vi "Controls-Loop.vi"(7 "CMD Notifier":refnum<notifier>, 8 "error in":errorcluster, 9 "Control Data Notifier":refnum<notifier>, 10 "Processed Data Notifier":refnum<notifier>, 11 "Message Queues":T2) -> (0 "error out":errorcluster)   [LabVIEW 2024]
uses:
  support/Message Queue/All Message Queues.ctl
  support/Message Queue/Message Cluster.ctl
  support/Control/Array Data Constant.ctl
  support/Control/Control Data Constant.ctl
  Controls State.ctl
  support/Control/DAQmx Container.ctl
  Sequence/Sequence Structure.ctl
  support/Control/BBControl Parameters.ctl
  support/Control/StreamCluster_TypeDef.ctl
  <vilib>/ErrorRing/Error Ring.xnode
  support/Message Queue/Message Queue.lvlib
  332b4253-326d-4d7b-9710-a01b345fab27.vi
  61c51413-b1d0-41cf-878e-839bc20d578b.vi
  c894b992-033a-4c8a-923e-e5ce24f73376.vi
panel:
  in  "Control Data":T1
  out "Loop-3 Iteration Clock (s) 2":dbl format="%10.8f"
  out "Loop-3 Iteration Counter 2":i32
  out "Loop-3 Iteration Counter":i32
  out "Loop-3 Iteration Clock (s)":dbl format="%10.8f"
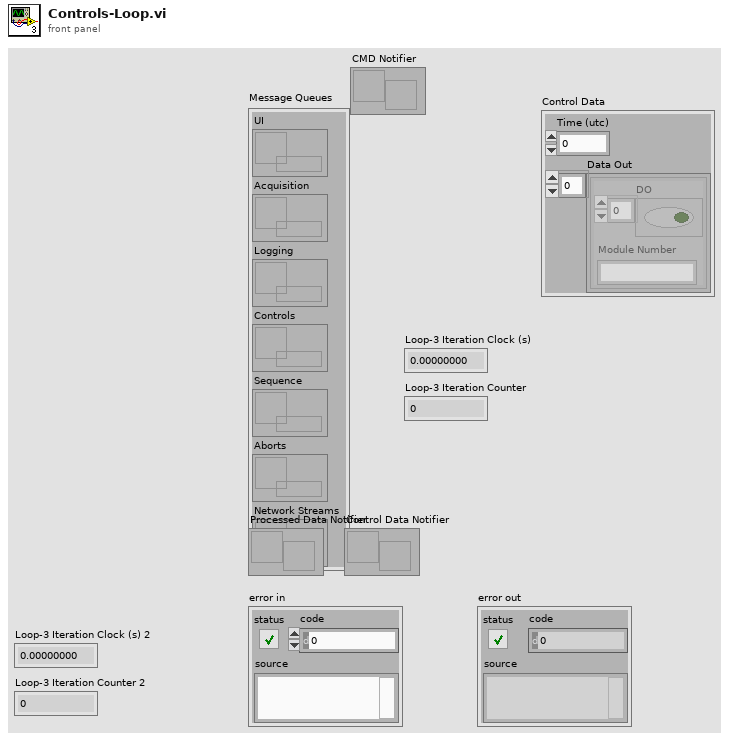
[diagram p1: front panel]
types:
  T1 = typedef "Control Data Constant.ctl" = cluster{"Time (utc)":ext, "Data Out":cluster{"DO":bool[], "Module Number":string}[]}
  T2 = typedef "Message Queue.lvlib/All Message Queues.ctl" = cluster{"UI":refnum<queue>, "Acquisition":refnum<queue>, "Logging":refnum<queue>, "Controls":refnum<queue>, "Sequence":refnum<queue>, "Aborts":refnum<queue>, "Network Streams":refnum<queue>}
  T3 = typedef "Controls State.ctl" = enum16{"Idle", "Control", "Sequencing", "Abort"}
  T4 = typedef "DAQmx Container.ctl" = cluster{"DAQmx Analog In":refnum<k21>, "DAQmx Digital In":refnum<k21>, "DAQmx Digital Out":refnum<k21>, "DAQmx Analog Out":refnum<k21>, "DAQmx 6343":refnum<k21>, "DAQmx IG-Sense":refnum<k21>, "DAQmx Thermo":refnum<k21>, "DAQmx Bridge":refnum<k21>, "DAQmx Trigger":refnum<k21>}
  T5 = typedef "LVDateTimeRec.ctl" = cluster{"fractional second":dbl, "second":i32, "minute":i32, "hour":i32, "day of month":i32, "month":i32, "year":i32, "day of week":i32, "day of year":i32, "DST":i32}
  T6 = typedef "BBControl Parameters.ctl" = cluster{"Sequence Delay (s)":dbl, "Sequence Duration (s)":dbl, "BBControl Criteria":cluster{"Channel Name":i32, "Comparison":u16, "Set":dbl, "Enabled":bool, "Valve Name":i32, "Upper":dbl, "Lower":dbl}[]}
  T7 = typedef "Sequence Structure.ctl" = cluster{"Sequence Controller":cluster{"Time (s)":dbl, "Enabled":bool, "Valve":u16[]}[], "Sequence Delay":dbl, "Sequence Duration":dbl}
  T8 = typedef "StreamCluster_TypeDef.ctl" = cluster{"DAQ":cluster{"ManagmentRate_Hz":i32, "StreamRate_Hz":i32, "StreamRate_ms":i32, "ManagmentRate_ms":i32, "refDesArray":cluster{"refDes-s":string[], "Module Number":string}[]}, "Modules":cluster{"Slot ID":i32, "Model Number":string, "Sample Rate s/S (Hz)":dbl, "Sensors":cluster{"refDes":string, "serialNumber":string, "modelNumber":string, "units":string, "balance":dbl, "sensitivity":dbl, "type":string, "inputTerminalConfiguration":string, "channelNumber":string, "taskName":string, "bridgeConfiguration":string, "excitationVoltage":dbl, "voltageExcitationSource":string, "nominalBridgeResistance":dbl, "firstElectricalValue":dbl, "secondElectricalValue":dbl, "firstPhysicalValue":dbl, "secondPhysicalValue":dbl, "electricalUnits":string}[]}[]}
  T9 = cluster{"refDes-s":string[], "Module Number":string}[]
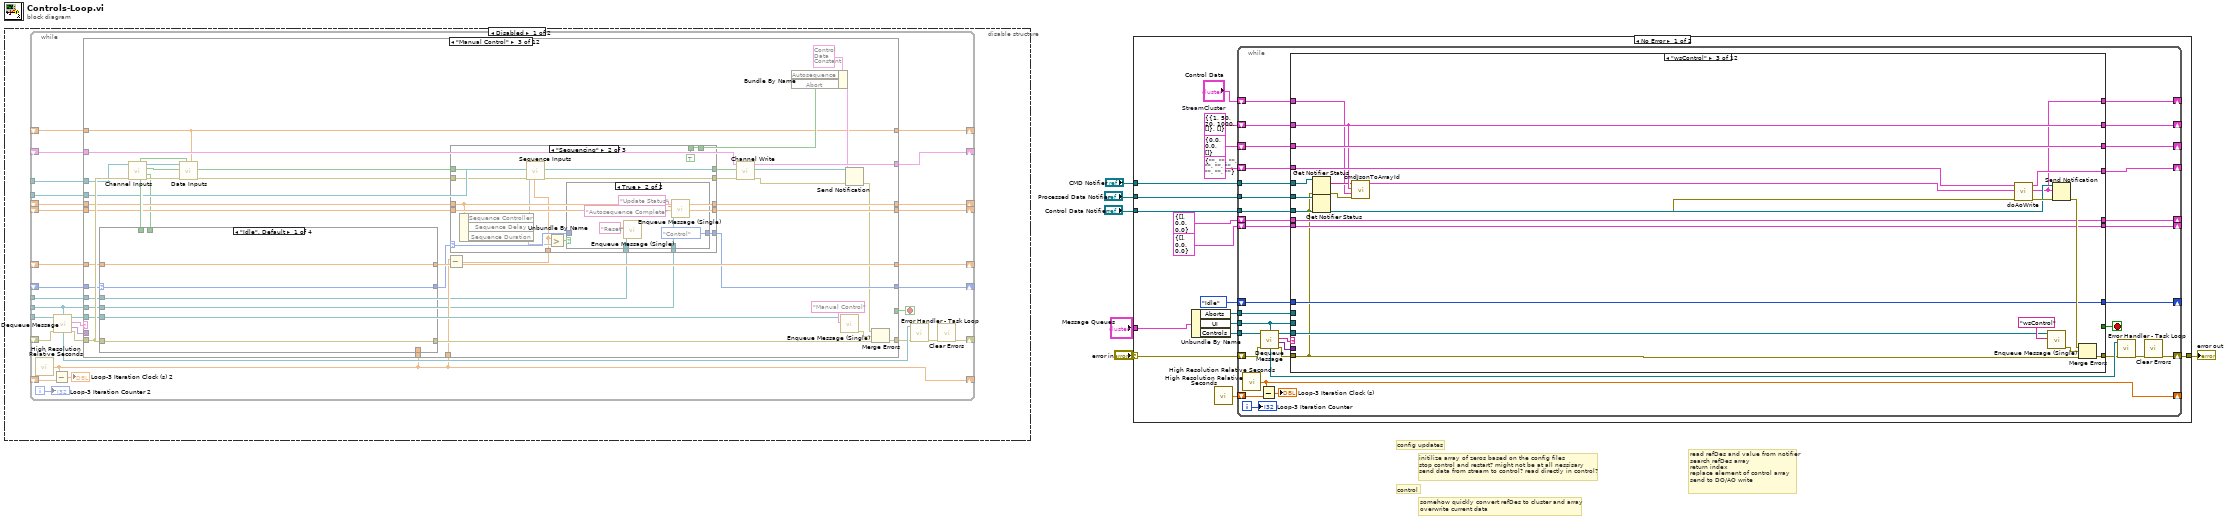
[diagram p0: block diagram]
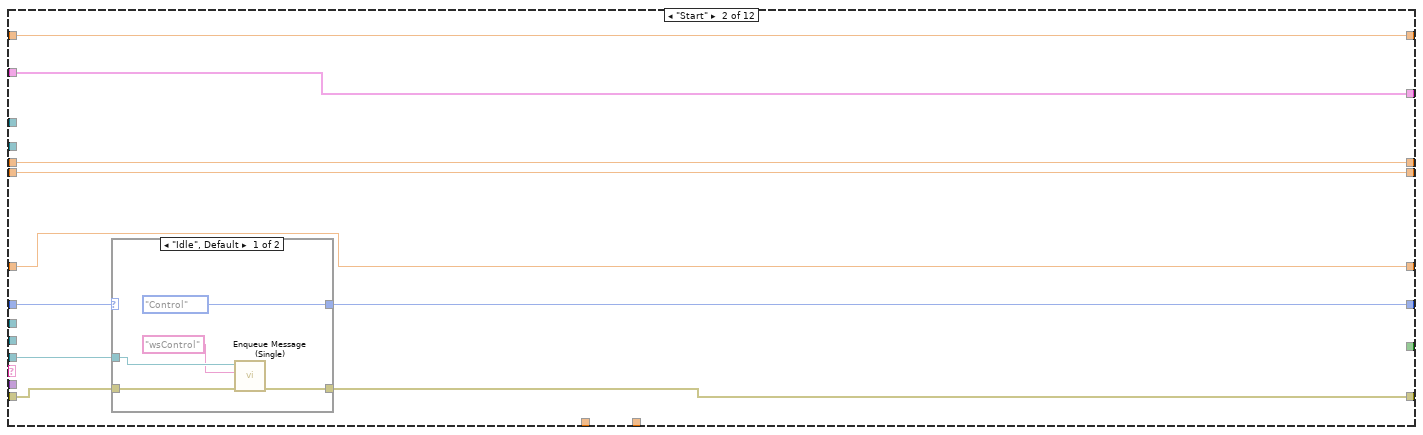
[diagram p3: hidden frame]
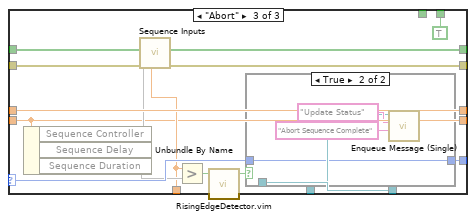
[diagram p7: hidden frame]
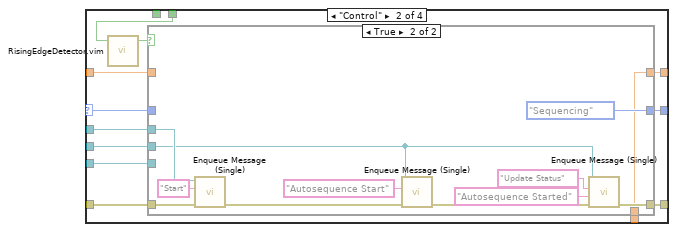
[diagram p9: hidden frame]
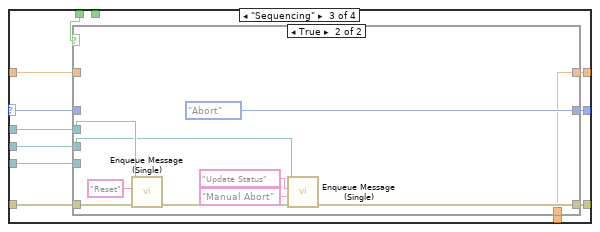
[diagram p11: hidden frame]
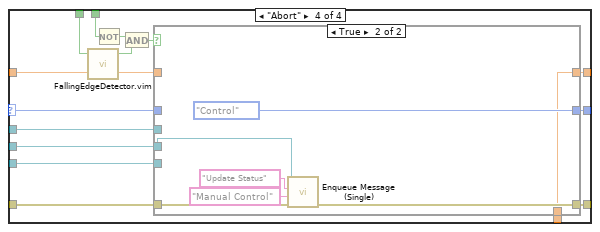
[diagram p13: hidden frame]
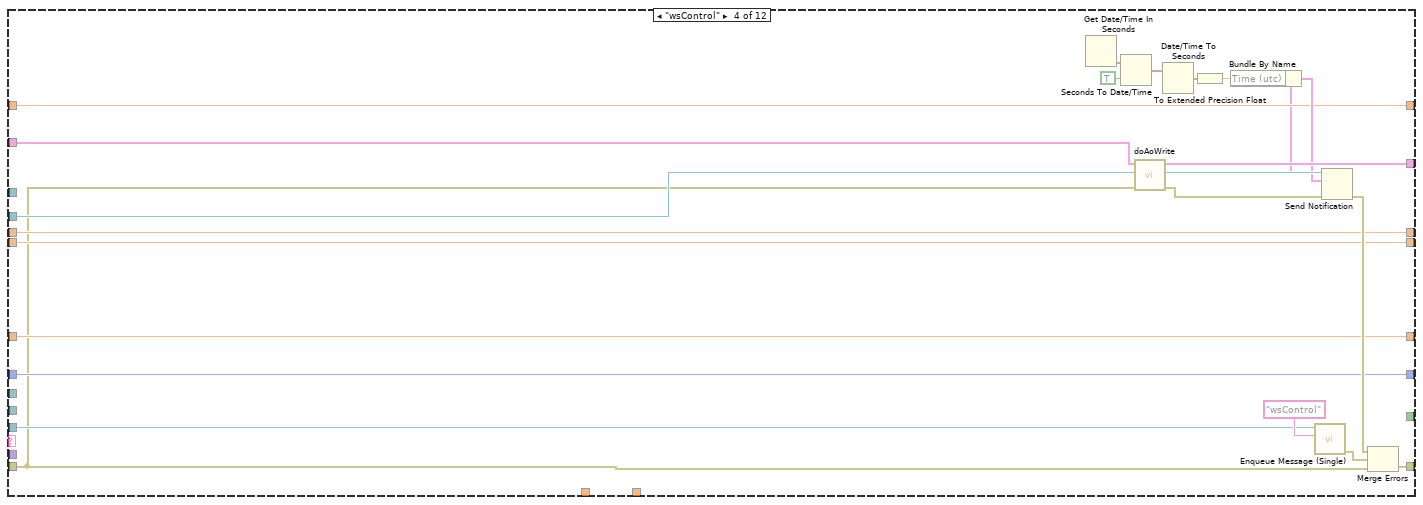
[diagram p15: hidden frame]
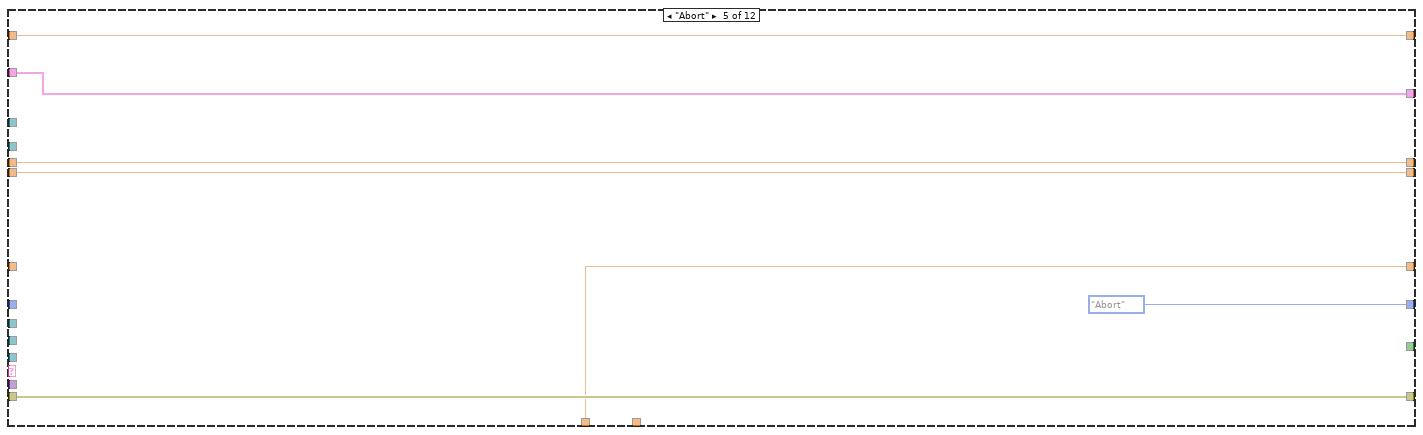
[diagram p16: hidden frame]
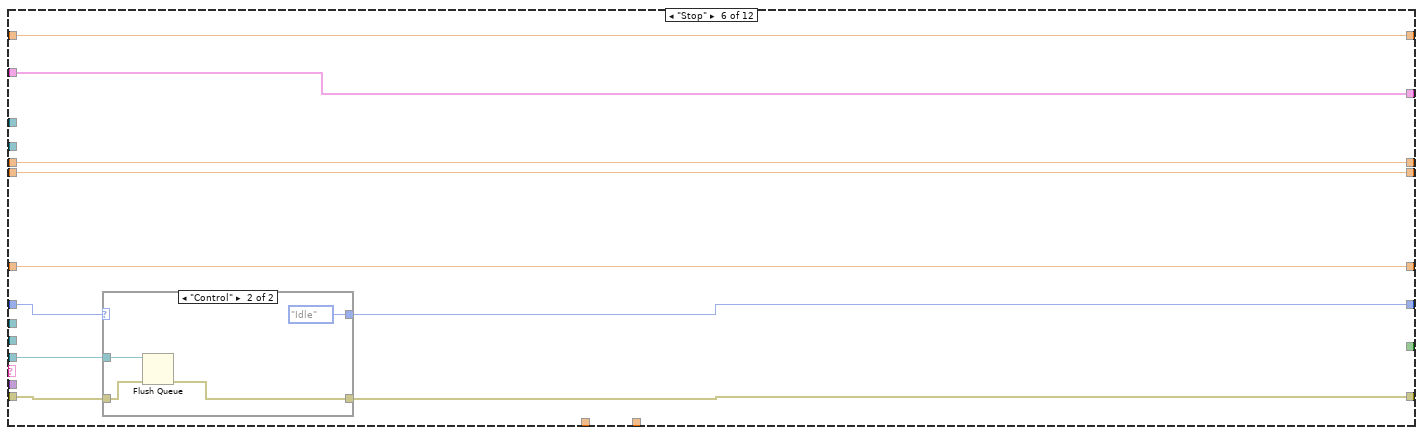
[diagram p17: hidden frame]
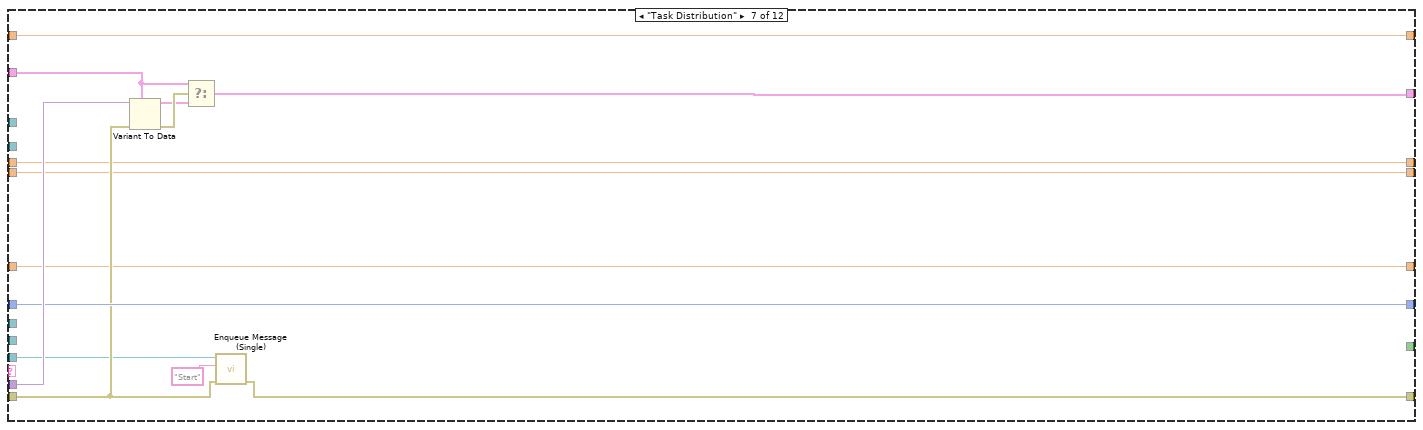
[diagram p19: hidden frame]
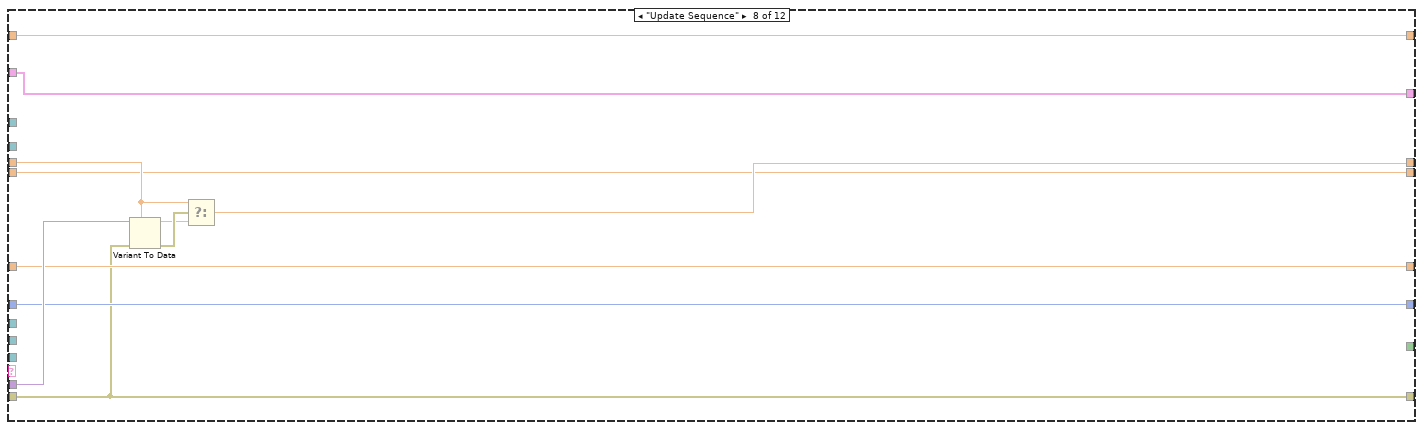
[diagram p20: hidden frame]
diagram:
  # "read refDes and value from notifier\nsearch refDes array\nreturn index\nreplace element of control array\nsend to DO/AO write"
  # "somehow quickly convert refDes to cluster and array\noverwrite current data"
  # "control"
  # "initilize array of zeros based on the config files \nstop control and restart? might not be at all nessisary\nsend data from stream to control? read directly in control?"
  # "config updates"
  n1 = disable-structure shown="Disabled" {
    frame Disabled {
      n2 = while {
        shift-right: [w9] -> _
        shift-left: _ -> [w34]
        tunnel: _ -> [w26]
        tunnel: _ -> [w35]
        shift-right: [w28] -> _
        shift-left: _ -> [w29]
        shift-right: [w16] -> _
        shift-left: _ -> [w24]
        tunnel: _ -> [w21]
        shift-right: [w19] -> _
        shift-left: _ -> [w20]
        tunnel: _ -> [w18]
        tunnel: _ -> [w17]
        shift-right: [w15] -> _
        shift-left: _ -> [w14]
        shift-right: [w12] -> _
        shift-left: _ -> [w13]
        shift-right: [w10] -> _
        shift-left: _ -> [w11]
        shift-right: [w7] -> _
        shift-left: _ -> [w8]
        i -> [w23]
        stop <- w27 stop-if-true
        n3 = call <vilib>:"High Resolution Relative Seconds.vi"() -> ("relative seconds"=w16:dbl)
        n4 = Subtract(x=w16, y=w24) -> (x-y=→"Loop-3 Iteration Clock (s) 2":dbl)
        n5 = call "Dequeue Message.vi"("error in (no error)"=w34, "Message Queue"=w35) -> ("error out"=w33:errorcluster, "Message Data"=w31:variant, "Message"=w30:string, "dup Message Queue"=w32:refnum<queue>)  [unwired: 6 in]
        n6 = case shown="\"Manual Control\"" w30 {
          selector: w30 -> [_ _ _ _ _ _ _ _ _ _ _ w345]
          tunnel: [w43 w49 w98 w249 w256 w263 w279 w289 w302 w313 w329 w346] -> w22
          tunnel: w33 -> [w43 w50 w101 w229 w256 w264 w281 w289 w302 w313 w332 _]
          tunnel: w32 -> [_ w51 w93 w245 _ w262 w280 _ _ _ w333 _]
          tunnel: w31 -> [_ _ _ _ _ _ w283 w295 w306 w317 _ _]
          tunnel: w29 -> [w42 w53 w99 w233 _ w266 w282 w294 w305 w316 w330 w344]
          tunnel: [w42 w52 w77 w233 Controls_State."Abort" ("Controls State") w265 w282 w294 w305 w316 w330 w344] -> w28
          tunnel: [w41 w48 w97 w248 w252 w261 w284 w290 w303 w314 w324 w343] -> w19
          tunnel: [_ _ _ _ _ _ _ _ _ _ TRUE _] -> w27
          tunnel: w26 -> [_ _ w72 _ _ _ _ _ _ _ w328 _]
          tunnel: w21 -> [_ _ w95 _ _ _ _ _ _ _ _ _]
          tunnel: w20 -> [w41 w48 w96 w247 w252 w261 w277 w290 w303 w314 w324 w343]
          tunnel: w18 -> [_ _ w65 _ _ _ _ _ _ _ _ _]
          tunnel: w17 -> [_ _ w69 w241 _ _ _ _ _ _ _ _]
          tunnel: w16 -> [_ _ w91 _ w253 _ _ _ _ _ _ _]
          tunnel: w16 -> [_ _ w88 _ _ _ _ _ _ _ _ _]
          tunnel: [w40 w47 w89 w232 w253 w260 w276 w293 w304 w315 w323 w342] -> w15
          tunnel: w14 -> [w40 w47 w90 w232 _ w260 w276 w293 w304 w315 w323 w342]
          tunnel: w13 -> [w39 w46 w75 w230 w254 w259 w275 w292 w299 w312 w322 w341]
          tunnel: [w39 w46 w74 w230 w254 w259 w275 w291 w299 w312 w322 w341] -> w12
          tunnel: w11 -> [w38 w45 w76 w231 w255 w258 w274 w288 w301 w311 w321 w340]
          tunnel: [w38 w45 w73 w231 w255 w258 w274 w288 w300 w311 w321 w340] -> w10
          tunnel: w8 -> [w37 w44 w61 w239 w250 w257 w273 w287 w298 w310 w320 w339]
          tunnel: [w37 w44 w61 w239 w250 w257 w273 w287 w298 w309 w320 w339] -> w7
          frame "Initialize" {
          }
          frame "Start" {
            n7 = case shown="\"Idle\", Default" w53 {
              selector: w53 -> [_ w60]
              tunnel: [Controls_State."Control" ("Controls State") w60] -> w52
              tunnel: w51 -> [w57 _]
              tunnel: w50 -> [w55 w59]
              tunnel: [w54 w59] -> w49
              frame "Idle", Default {
                n8 = call "Enqueue Message (Single).vi"("error in (no error)"=w55, "Message"="wsControl", "Message Queue"=w57) -> ("error out"=w54:errorcluster)  [unwired: 7 in, 1 out]
              }
              frame "Control" {
              }
            }
          }
          frame "Manual Control" {
            n9 = call "Channel Inputs.vi"("Data Notifier"=w95, "error in"=w101) -> ("BangBang\nArm out"=w62:bool, "Data Notifier out"=w85:refnum<notifier>, "Actuation Array"=w84:bool[], "Auto-sequence"=w66:bool, "Abort"=w87:bool, "error out"=w86:errorcluster)  [unwired: 8 in]
            n10 = case shown="\"Idle\", Default" w99 {
              selector: w99 -> [w151 w157 w184 w211]
              tunnel: w93 -> [_ w159 w186 w213]
              tunnel: w101 -> [w150 w158 w185 w212]
              tunnel: [w150 w162 w188 w216] -> w100
              tunnel: [w151 w163 w189 w217] -> w83
              tunnel: w72 -> [_ w160 w187 w214]
              tunnel: w65 -> [_ w161 w179 w215]
              tunnel: w66 -> [_ w153 _ w207]
              tunnel: w87 -> [_ _ w183 w204]
              tunnel: w91 -> [_ w156 w182 w210]
              tunnel: [w149 w155 w181 w209] -> w89
              tunnel: w90 -> [w149 w154 w180 w208]
              frame "Idle", Default {
              }
              frame "Control" {
                n11 = call "RisingEdgeDetector.vim"("Data"=w153) -> ("Edge?"=w152:bool)  [unwired: 4 in]
                n12 = case shown="True" w152 {
                  tunnel: [w166 Controls_State."Sequencing" ("Controls State")] -> w163
                  tunnel: w161 -> [_ w177]
                  tunnel: w158 -> [w165 w175]
                  tunnel: [w165 w172] -> w162
                  tunnel: w160 -> [_ w169]
                  tunnel: w159 -> [_ _]
                  tunnel: w157 -> [w166 _]
                  tunnel: [w164 w171] -> w155
                  tunnel: w156 -> [_ w171]
                  tunnel: w154 -> [w164 _]
                  frame False {
                  }
                  frame True {
                    n13 = call "Enqueue Message (Single).vi"("error in (no error)"=w175, "Message"="Start", "Message Queue"=w177) -> ("error out"=w167:errorcluster)  [unwired: 7 in, 1 out]
                    n14 = call "Enqueue Message (Single).vi"("error in (no error)"=w167, "Message"="Autosequence Start", "Message Queue"=w169) -> ("error out"=w168:errorcluster)  [unwired: 7 in, 1 out]
                    n15 = call "Enqueue Message (Single).vi"("error in (no error)"=w168, "Message Data"="Autosequence Started", "Message"="Update Status", "Message Queue"=w169) -> ("error out"=w172:errorcluster)  [unwired: 6 in, 1 out]
                  }
                }
              }
              frame "Sequencing" {
                n16 = case shown="True" w183 {
                  tunnel: [w192 Controls_State."Abort" ("Controls State")] -> w189
                  tunnel: w179 -> [_ w201]
                  tunnel: w185 -> [w191 w200]
                  tunnel: [w191 w196] -> w188
                  tunnel: w187 -> [_ w195]
                  tunnel: w186 -> [_ _]
                  tunnel: w184 -> [w192 _]
                  tunnel: w182 -> [_ w193]
                  tunnel: [w190 w193] -> w181
                  tunnel: w180 -> [w190 _]
                  frame False {
                  }
                  frame True {
                    n17 = call "Enqueue Message (Single).vi"("error in (no error)"=w200, "Message"="Reset", "Message Queue"=w201) -> ("error out"=w197:errorcluster)  [unwired: 7 in, 1 out]
                    n18 = call "Enqueue Message (Single).vi"("error in (no error)"=w197, "Message Data"="Manual Abort", "Message"="Update Status", "Message Queue"=w195) -> ("error out"=w196:errorcluster)  [unwired: 6 in, 1 out]
                  }
                }
              }
              frame "Abort" {
                n19 = call "FallingEdgeDetector.vim"("Data"=w204) -> ("Edge?"=w203:bool)  [unwired: 4 in]
                n20 = Not(x=w207) -> (.not. x?=w205:bool)
                n21 = And(x=w205, y=w203) -> (x .and. y?=w206:bool)
                n22 = case shown="True" w206 {
                  tunnel: [w220 Controls_State."Control" ("Controls State")] -> w217
                  tunnel: w215 -> [_ _]
                  tunnel: w212 -> [w219 w221]
                  tunnel: [w219 w224] -> w216
                  tunnel: w214 -> [_ w223]
                  tunnel: w213 -> [_ _]
                  tunnel: w211 -> [w220 _]
                  tunnel: w210 -> [_ w222]
                  tunnel: [w218 w222] -> w209
                  tunnel: w208 -> [w218 _]
                  frame False {
                  }
                  frame True {
                    n23 = call "Enqueue Message (Single).vi"("error in (no error)"=w221, "Message Data"="Manual Control", "Message"="Update Status", "Message Queue"=w223) -> ("error out"=w224:errorcluster)  [unwired: 6 in, 1 out]
                  }
                }
              }
            }
            n24 = call "Data Inputs.vi"("BBControl Parameters"=w61, "Arm"=w62, "error in"=w86, "Actuation Array in"=w84, "Data Notifier"=w85) -> ("error out"=w82:errorcluster, "Actuation Array out"=w80:bool[])  [unwired: 4 in, 1 out]
            n25 = Subtract(x=w88, y=w89) -> (x-y=w78:dbl)
            n26 = case shown="\"Sequencing\"" w83 {
              selector: w83 -> [w104 w120 w142]
              tunnel: w82 -> [w106 w115 w138]
              tunnel: [w106 w114 w137] -> w81
              tunnel: w80 -> [w105 w112 w135]
              tunnel: [w105 w111 w134] -> w79
              tunnel: w78 -> [_ w113 w136]
              tunnel: [w104 w119 w141] -> w77
              tunnel: w76 -> [w102 w118 w132]
              tunnel: w75 -> [w103 w117 w140]
              tunnel: [w103 w117 w140] -> w74
              tunnel: [w102 w118 w132] -> w73
              tunnel: w72 -> [_ w109 w131]
              tunnel: [_ TRUE _] -> w64
              tunnel: w65 -> [_ w107 _]
              tunnel: [_ _ TRUE] -> w63
              frame Default {
              }
              frame "Sequencing" {
                n27 = Unbundle By Name(w117) -> ("Sequence Controller"=w110, "Sequence Duration"=w116)  [unwired: 1 out]
                n28 = call "Sequence Inputs.vi"("Time In"=w113, "error in"=w115, "Actuation Array in"=w112, "Sequence"=w110) -> ("error out"=w114:errorcluster, "Actuation Array out"=w111:bool[])  [unwired: 6 in]
                n29 = Greater?(x=w113, y=w116) -> (0:w121:bool)
                n30 = case shown="True" w121 {
                  tunnel: w120 -> [w122 _]
                  tunnel: [w122 Controls_State."Control" ("Controls State")] -> w119
                  tunnel: w109 -> [_ w125]
                  tunnel: w107 -> [_ w123]
                  frame False {
                  }
                  frame True {
                    n31 = call "Enqueue Message (Single).vi"("Message"="Reset", "Message Queue"=w123) -> ()  [unwired: 8 in, 2 out]
                    n32 = call "Enqueue Message (Single).vi"("Message Data"="Autosequence Complete", "Message"="Update Status", "Message Queue"=w125) -> ()  [unwired: 7 in, 2 out]
                  }
                }
              }
              frame "Abort" {
                n33 = Unbundle By Name(w132) -> ("Sequence Controller"=w133, "Sequence Duration"=w139)  [unwired: 1 out]
                n34 = call "Sequence Inputs.vi"("Time In"=w136, "error in"=w138, "Actuation Array in"=w135, "Sequence"=w133) -> ("error out"=w137:errorcluster, "Actuation Array out"=w134:bool[])  [unwired: 6 in]
                n35 = Greater?(x=w136, y=w139) -> (0:w143:bool)
                n36 = call "RisingEdgeDetector.vim"("Data"=w143) -> ("Edge?"=w130:bool)  [unwired: 4 in]
                n37 = case shown="True" w130 {
                  tunnel: w142 -> [w144 w145]
                  tunnel: [w144 w145] -> w141
                  tunnel: w131 -> [_ w146]
                  frame False {
                  }
                  frame True {
                    n38 = call "Enqueue Message (Single).vi"("Message Data"="Abort Sequence Complete", "Message"="Update Status", "Message Queue"=w146) -> ()  [unwired: 7 in, 2 out]
                  }
                }
              }
            }
            n39 = call "Channel Write.vi"("error in"=w81, "Actuation Array"=w79, "DAQmx Container In"=w96) -> ("error out"=w71:errorcluster, "DAQmx Container Out"=w97:T4)  [unwired: 6 in, 1 out]
            n40 = Bundle By Name(cluster=T1 {"Time (utc)"=0.0, "Data Out"=[]} ("notification"), "Autosequence"=w64, "Abort"=w63) -> (w67:T1)
            n41 = call "Enqueue Message (Single).vi"("Message"="Manual Control", "Message Queue"=w93) -> ("error out"=w92:errorcluster)  [unwired: 8 in, 1 out]
            n42 = Send Notification(notification=w67, notifier=w69, error in (no error)=w71) -> (error out=w70:errorcluster)  [unwired: 1 out]
            n43 = Merge Errors(w70, w92, w100) -> (w98:errorcluster)
          }
          frame "wsControl" {
            n44 = Get Date/Time In Seconds() -> (seconds since 1Jan1904=w237:timestamp)
            n45 = Seconds To Date/Time(time stamp (now)=w237, to UTC (F)=TRUE) -> (date time rec=w238:T5)
            n46 = call "doAoWrite.vi"("error in"=w229, "DAQmx Container In"=w247) -> ("error out"=w243:errorcluster, "Control Data"=w228:T1, "DAQmx Container Out"=w248:T4)  [unwired: 7 in]
            n47 = Date/Time To Seconds(2:w238) -> (0:w235:timestamp)  [unwired: 1 in]
            n48 = To Extended Precision Float(1:w235) -> (0:w234:ext)
            n49 = Bundle By Name(cluster=w228, "Time (utc)"=w234) -> (w240:T1)
            n50 = call "Enqueue Message (Single).vi"("Message"="wsControl", "Message Queue"=w245) -> ("error out"=w244:errorcluster)  [unwired: 8 in, 1 out]
            n51 = Send Notification(notification=w240, notifier=w241, error in (no error)=w243) -> (error out=w242:errorcluster)  [unwired: 1 out]
            n52 = Merge Errors(w242, w244, w229) -> (w249:errorcluster)
          }
          frame "Abort" {
          }
          frame "Stop" {
            n53 = case shown="\"Control\"" w266 {
              selector: w266 -> [w268 _]
              tunnel: [w268 Controls_State."Idle" ("Controls State")] -> w265
              tunnel: w264 -> [w267 w270]
              tunnel: [w267 w269] -> w263
              tunnel: w262 -> [_ w271]
              frame "Idle", Default {
              }
              frame "Control" {
                n54 = Flush Queue(queue=w271, error in (no error)=w270) -> (error out=w269:errorcluster)  [unwired: 2 out]
              }
            }
          }
          frame "Task Distribution" {
            n55 = Variant To Data(error in=w281, type=w277, Variant=w283) -> (data=w285:T4, error out=w286:errorcluster)
            n56 = Select(t=w277, s=w286, f=w285) -> (s? t:f=w284:T4)
            n57 = call "Enqueue Message (Single).vi"("error in (no error)"=w281, "Message"="Start", "Message Queue"=w280) -> ("error out"=w279:errorcluster)  [unwired: 7 in, 1 out]
          }
          frame "Update Sequence" {
            n58 = Variant To Data(error in=w289, type=w292, Variant=w295) -> (data=w296:dbl, error out=w297:errorcluster)
            n59 = Select(t=w292, s=w297, f=w296) -> (s? t:f=w291:dbl)
          }
          frame "Update AbortSequence" {
            n60 = Variant To Data(error in=w302, type=w301, Variant=w306) -> (data=w307:dbl, error out=w308:errorcluster)
            n61 = Select(t=w301, s=w308, f=w307) -> (s? t:f=w300:dbl)
          }
          frame "Update BBControl" {
            n62 = Variant To Data(error in=w313, type=w310, Variant=w317) -> (data=w318:dbl, error out=w319:errorcluster)
            n63 = Select(t=w310, s=w319, f=w318) -> (s? t:f=w309:dbl)
          }
          frame "Leave" {
            n64 = Release Queue(queue=w333, error in (no error)=w332) -> (error out=w326:errorcluster)  [unwired: 1 in, 2 out]
            n65 = Get Queue Status(queue=w328) -> (queue out=w327:refnum<queue>, error out=w325:errorcluster)  [unwired: 2 in, 6 out]
            n66 = case shown="No Error" w325 {
              tunnel: [w336 w338] -> w329
              tunnel: w327 -> [w335 _]
              tunnel: w326 -> [w334 w338]
              frame No Error {
                n67 = call "Enqueue Message (Single).vi"("error in (no error)"=w334, "Message"="Leave", "Message Queue"=w335) -> ("error out"=w336:errorcluster)  [unwired: 7 in, 1 out]
              }
              frame Error {
              }
            }
          }
          frame Default {
            n68 = xnode "Error Ring"("parameter 0"=w345) -> ("error out"=w346:errorcluster)
          }
        }
        n69 = call "Error Handler - Task Loop.vi"("error in (no error)"=w22, "Message Queue"=w26) -> ("dup error in"=w36:errorcluster)  [unwired: 8 in, 1 out]
        n70 = call <vilib>:"Clear Errors.vi"("error in (no error)"=w36) -> ("error out"=w9:errorcluster)  [unwired: 5 in, 1 out]
        "Loop-3 Iteration Counter 2" <- w23
      }
    }
    frame Enabled {
    }
  }
  n71 = case shown="No Error" "error in" {
    selector: "error in" -> [w368 w588]
    tunnel: [w367 w588] -> w5
    tunnel: "Message Queues" -> [w366 _]
    tunnel: "Processed Data Notifier" -> [w361 _]
    tunnel: "Control Data Notifier" -> [w358 _]
    tunnel: "CMD Notifier" -> [w354 _]
    frame No Error {
      w353 = T8 {"DAQ"={"ManagmentRate_Hz"=1, "StreamRate_Hz"=50, "StreamRate_ms"=20, "ManagmentRate_ms"=1000, "refDesArray"=[]}, "Modules"=[]}  # StreamCluster
      n72 = Unbundle By Name(w366) -> ("Aborts"=w359:refnum<queue>, "UI"=w365:refnum<queue>, "Controls"=w364:refnum<queue>)
      n73 = call <vilib>:"High Resolution Relative Seconds.vi"() -> ("relative seconds"=w362:dbl)
      n74 = while {
        shift-right: [w377] -> w367
        shift-left: w368 -> [w399]
        tunnel: w365 -> [w391]
        tunnel: w364 -> [w400]
        shift-right: [w393] -> _
        shift-left: Controls_State."Idle" ("Controls State") -> [w394]
        shift-right: [w374] -> _
        shift-left: w362 -> [w389]
        tunnel: w361 -> [w386]
        shift-right: [w384] -> _
        shift-left: T4 {"DAQmx Analog In"="", "DAQmx Digital In"="", "DAQmx Digital Out"="", "DAQmx Analog Out"="", "DAQmx 6343"="", "DAQmx IG-Sense"="", "DAQmx Thermo"="", "DAQmx Bridge"="", "DAQmx Trigger"=""} ("DAQmx Container") -> [w385]
        tunnel: w359 -> [w383]
        tunnel: w358 -> [w382]
        shift-right: [w380] -> _
        shift-left: T7 {"Sequence Controller"=[], "Sequence Delay"=0.0, "Sequence Duration"=0.0} ("Sequence Conditions") -> [w381]
        shift-right: [w378] -> _
        shift-left: T7 {"Sequence Controller"=[], "Sequence Delay"=0.0, "Sequence Duration"=0.0} ("Sequence Conditions") -> [w379]
        shift-right: [w375] -> _
        shift-left: T6 {"Sequence Delay (s)"=0.0, "Sequence Duration (s)"=0.0, "BBControl Criteria"=[]} ("BBControl Parameters") -> [w376]
        tunnel: w354 -> [w373]
        shift-right: [w371] -> _
        shift-left: w353 -> [w372]
        shift-right: [w370] -> _
        shift-left: "Control Data" -> [w369]
        i -> [w388]
        stop <- w392 stop-if-true
        n75 = call <vilib>:"High Resolution Relative Seconds.vi"() -> ("relative seconds"=w374:dbl)
        n76 = Subtract(x=w374, y=w389) -> (x-y=→"Loop-3 Iteration Clock (s)":dbl)
        n77 = call "Dequeue Message.vi"("error in (no error)"=w399, "Message Queue"=w400) -> ("error out"=w398:errorcluster, "Message Data"=w396:variant, "Message"=w395:string, "dup Message Queue"=w397:refnum<queue>)  [unwired: 6 in]
        n78 = case shown="\"wsControl\"" w395 {
          selector: w395 -> [_ _ _ _ _ _ _ _ _ _ _ w581]
          tunnel: [w409 w416 w450 w458 w466 w483 w495 w509 w521 w541 w564 w582] -> w387
          tunnel: w398 -> [w409 w417 w435 w458 w467 w485 w495 w509 w521 w541 w567 _]
          tunnel: w397 -> [_ w418 w446 _ w465 w484 _ _ _ _ w568 _]
          tunnel: w396 -> [_ _ _ _ _ w487 w500 w512 w524 w544 _ _]
          tunnel: w394 -> [w408 w420 w440 _ w469 w486 w499 w511 w523 w543 w565 w580]
          tunnel: [w408 w419 w440 Controls_State."Abort" ("Controls State") w468 w486 w499 w511 w523 w543 w565 w580] -> w393
          tunnel: [w407 w415 w449 w455 w464 w488 w496 w510 w522 w542 w559 w579] -> w384
          tunnel: [_ _ _ _ _ _ _ _ _ _ TRUE _] -> w392
          tunnel: w391 -> [_ _ _ _ _ _ _ _ _ _ w563 _]
          tunnel: w386 -> [_ _ w437 _ _ _ _ _ _ _ _ _]
          tunnel: w385 -> [w407 w415 w448 w455 w464 w481 w496 w510 w522 w542 w559 w579]
          tunnel: w383 -> [_ _ _ _ _ _ _ _ _ _ _ _]
          tunnel: w382 -> [_ _ w442 _ _ _ _ _ _ _ _ _]
          tunnel: w381 -> [w406 w414 w438 w456 w463 w480 w498 w506 w520 w540 w558 w578]
          tunnel: [w406 w414 w438 w456 w463 w480 w497 w506 w520 w540 w558 w578] -> w380
          tunnel: w379 -> [w405 w413 w439 w457 w462 w479 w494 w508 w519 w539 w557 w577]
          tunnel: [w405 w413 w439 w457 w462 w479 w494 w507 w519 w539 w557 w577] -> w378
          tunnel: w376 -> [w404 w412 w441 w453 w461 w478 w493 w505 w518 w538 w556 w576]
          tunnel: [w404 w412 w441 w453 w461 w478 w493 w505 w517 w538 w556 w576] -> w375
          tunnel: w373 -> [_ _ w434 _ _ _ _ _ _ _ _ _]
          tunnel: w372 -> [w403 w411 w433 w452 w460 w477 w492 w504 w516 w537 w555 w575]
          tunnel: [w403 w411 w433 w452 w460 w477 w492 w504 w516 w536 w555 w575] -> w371
          tunnel: [w402 w410 w428 w451 w459 w476 w491 w503 w515 w534 w554 w574] -> w370
          tunnel: w369 -> [w402 w410 w430 w451 w459 w476 w491 w503 w515 w532 w554 w574]
          frame "Initialize" {
          }
          frame "Start" {
            n79 = case shown="\"Idle\", Default" w420 {
              selector: w420 -> [_ w427]
              tunnel: [Controls_State."Control" ("Controls State") w427] -> w419
              tunnel: w418 -> [w424 _]
              tunnel: w417 -> [w422 w426]
              tunnel: [w421 w426] -> w416
              frame "Idle", Default {
                n80 = call "Enqueue Message (Single).vi"("error in (no error)"=w422, "Message"="wsControl", "Message Queue"=w424) -> ("error out"=w421:errorcluster)  [unwired: 7 in, 1 out]
              }
              frame "Control" {
              }
            }
          }
          frame "wsControl" {
            n81 = Get Notifier Status(notifier=w434, error in (no error)=w435) -> (current notification=w432:string, error out=w431:errorcluster)  [unwired: 3 out]
            n82 = Get Notifier Status(notifier=w437, error in (no error)=w435) -> (error out=w436:errorcluster)  [unwired: 4 out]
            n83 = call "cmdJsonToArrayId.vi"("error in"=w431, "Control Data"=w430, "StreamCluster"=w433, "JSON in"=w432) -> ("Control Data"=w429:T1)  [unwired: 6 in, 1 out]
            n84 = call "doAoWrite.vi"("error in"=w436, "Control Data"=w429, "DAQmx Container In"=w448) -> ("error out"=w444:errorcluster, "Control Data"=w428:T1, "DAQmx Container Out"=w449:T4)  [unwired: 6 in]
            n85 = call "Enqueue Message (Single).vi"("Message"="wsControl", "Message Queue"=w446) -> ("error out"=w445:errorcluster)  [unwired: 8 in, 1 out]
            n86 = Send Notification(notification=w428, notifier=w442, error in (no error)=w444) -> (error out=w443:errorcluster)  [unwired: 1 out]
            n87 = Merge Errors(w443, w445, w435) -> (w450:errorcluster)
          }
          frame "Abort" {
          }
          frame "Stop" {
            n88 = case shown="\"Control\"" w469 {
              selector: w469 -> [w471 _]
              tunnel: [w471 Controls_State."Idle" ("Controls State")] -> w468
              tunnel: w467 -> [w470 w473]
              tunnel: [w470 w472] -> w466
              tunnel: w465 -> [_ w474]
              frame "Idle", Default {
              }
              frame "Control" {
                n89 = Flush Queue(queue=w474, error in (no error)=w473) -> (error out=w472:errorcluster)  [unwired: 2 out]
              }
            }
          }
          frame "Task Distribution" {
            n90 = Variant To Data(error in=w485, type=w481, Variant=w487) -> (data=w489:T4, error out=w490:errorcluster)
            n91 = Select(t=w481, s=w490, f=w489) -> (s? t:f=w488:T4)
            n92 = call "Enqueue Message (Single).vi"("error in (no error)"=w485, "Message"="Start", "Message Queue"=w484) -> ("error out"=w483:errorcluster)  [unwired: 7 in, 1 out]
          }
          frame "Update Sequence" {
            n93 = Variant To Data(error in=w495, type=w498, Variant=w500) -> (data=w501:T7, error out=w502:errorcluster)
            n94 = Select(t=w498, s=w502, f=w501) -> (s? t:f=w497:T7)
          }
          frame "Update AbortSequence" {
            n95 = Variant To Data(error in=w509, type=w508, Variant=w512) -> (data=w513:T7, error out=w514:errorcluster)
            n96 = Select(t=w508, s=w514, f=w513) -> (s? t:f=w507:T7)
          }
          frame "Update BBControl" {
            n97 = Variant To Data(error in=w521, type=w518, Variant=w524) -> (data=w525:T6, error out=w526:errorcluster)
            n98 = Select(t=w518, s=w526, f=w525) -> (s? t:f=w517:T6)
          }
          frame "Update Config" {
            n99 = Variant To Data(error in=w541, type=w537, Variant=w544) -> (data=w545:T8, error out=w535:errorcluster)
            n100 = Select(t=w537, s=w535, f=w545) -> (s? t:f=w536:T8)
            n101 = Unbundle By Name(w536) -> ("DAQ.refDesArray"=w529:T9)
            n102 = Array Size(array=w529) -> (size(s)=w530:i32)
            n103 = Unbundle By Name(w532) -> ("Data Out"=w528:cluster{"DO":bool[], "Module Number":string}[])
            n104 = Index Array(array=w528) -> (element=w527:cluster{"DO":bool[], "Module Number":string})  [unwired: 1 in]
            n105 = for {
              N: w530 -> [_]
              tunnel: w529 -> [w551] mode=indexing
              tunnel: w527 -> [w549]
              tunnel: [w547] -> w533 mode=indexing
              n106 = Unbundle(w551) -> ("refDes-s"=w550:string[], "Module Number"=w546:string)
              n107 = Array Size(array=w550) -> (size(s)=w552:i32)
              n108 = Initialize Array(FALSE, w552) -> (w548:bool[])
              n109 = Bundle By Name(cluster=w549, "DO"=w548, "Module Number"=w546) -> (w547:cluster{"DO":bool[], "Module Number":string})
            }
            n110 = Bundle By Name(cluster=w532, "Data Out"=w533) -> (w531:T1)
            n111 = Select(t=w532, s=w535, f=w531) -> (s? t:f=w534:T1)
          }
          frame "Leave" {
            n112 = Release Queue(queue=w568, error in (no error)=w567) -> (error out=w561:errorcluster)  [unwired: 1 in, 2 out]
            n113 = Get Queue Status(queue=w563) -> (queue out=w562:refnum<queue>, error out=w560:errorcluster)  [unwired: 2 in, 6 out]
            n114 = case shown="No Error" w560 {
              tunnel: [w571 w573] -> w564
              tunnel: w562 -> [w570 _]
              tunnel: w561 -> [w569 w573]
              frame No Error {
                n115 = call "Enqueue Message (Single).vi"("error in (no error)"=w569, "Message"="Leave", "Message Queue"=w570) -> ("error out"=w571:errorcluster)  [unwired: 7 in, 1 out]
              }
              frame Error {
              }
            }
          }
          frame Default {
            n116 = xnode "Error Ring"("parameter 0"=w581) -> ("error out"=w582:errorcluster)
          }
        }
        n117 = call "Error Handler - Task Loop.vi"("error in (no error)"=w387, "Message Queue"=w391) -> ("dup error in"=w401:errorcluster)  [unwired: 8 in, 1 out]
        n118 = call <vilib>:"Clear Errors.vi"("error in (no error)"=w401) -> ("error out"=w377:errorcluster)  [unwired: 5 in, 1 out]
        "Loop-3 Iteration Counter" <- w388
      }
    }
    frame Error {
    }
  }
  "error out" <- w5
